vi "TypeDefExample.vi"() -> ()   [LabVIEW 2019]
uses:
  Employee.ctl
panel:
  in  "Employee 6":T1
  in  "Employee 5":T1
  in  "Employee 4":T1
  in  "Employee 3":T1
  in  "Employee 2":T1
  in  "Employee":T1
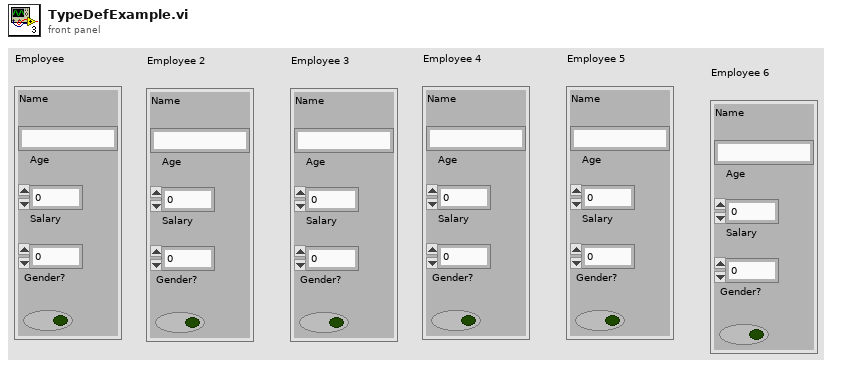
[diagram p1: front panel]
types:
  T1 = typedef "Employee.ctl" = cluster{"Name":string, "Age":u8, "Salary":u16, "Gender?":bool}
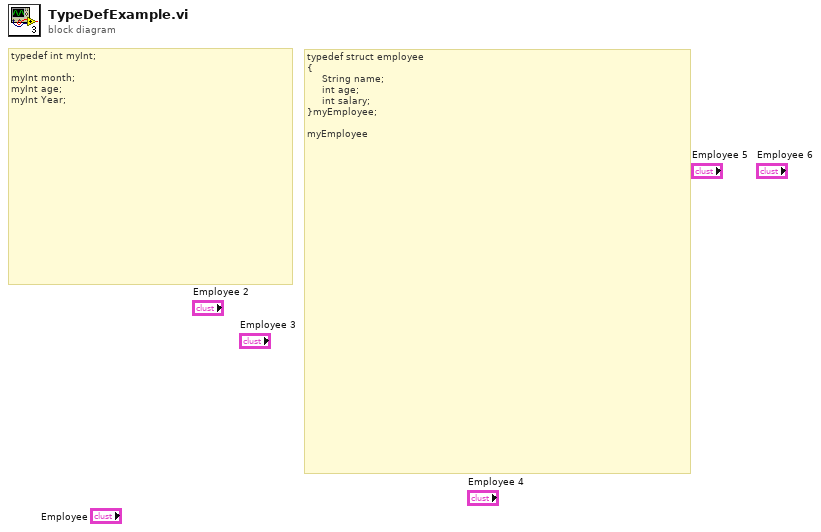
[diagram p0: block diagram]
diagram:
  # "typedef struct employee\n{\n     String name;\n     int age;\n     int salary;\n}myEmployee;\n\nmyEmployee"
  # "typedef int myInt;\n\nmyInt month;\nmyInt age;\nmyInt Year;"
